vi "Open FPGA Reference.vi"(0 "resource name":T1, 5 "Bitfile Name":string="MicroBlaze_lwIP-Test-Harness.lvbitx", 11 "Error In":errorcluster) -> (4 "FPGA VI Reference Out":refnum<k20>, 15 "error out":errorcluster)   [LabVIEW 2017, in "My Network Host v1.lvlib"]
uses:
  My Network Host v1.lvlib
  <vilib>/userdefined/Silver/nirio_resource_slv.ctl
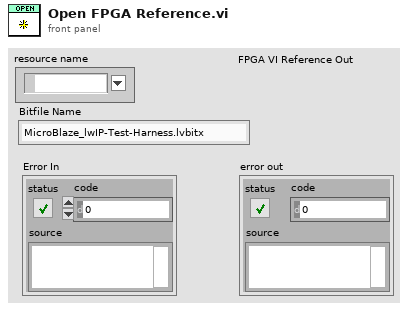
[diagram p1: front panel]
types:
  T1 = typedef "nirio_resource_slv.ctl" = tag
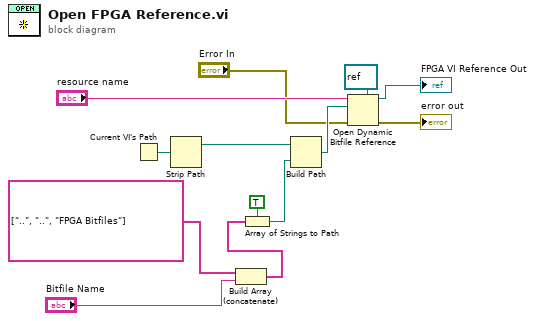
[diagram p0: block diagram]
diagram:
  n1 = Current VI's Path() -> (path=w9:path)
  n2 = Strip Path(path=w9) -> (stripped path=w8:path)  [unwired: 1 out]
  n3 = Build Array (concatenate)(string[] ["..", "..", "FPGA Bitfiles"] ("array of strings"), "Bitfile Name") -> (w2:string[])
  n4 = Array of Strings to Path(0:w2, 1:TRUE ("relative")) -> (2:w6:path)
  n5 = Build Path(base path=w8, name or relative path=w6) -> (appended path=w5:path)
  n6 = Open Dynamic Bitfile Reference(0:"resource name", 1:w5, 3:"Error In", 4:refnum<k20> refnum ("FPGA VI Reference Out")) -> (5:→"FPGA VI Reference Out":refnum<k20>, 8:→"error out":errorcluster)  [unwired: 1 in]
